vi "uTTA_Reset.vi"(4 "error in":errorcluster, 7 "uTTA Port":refnum<visa-resource-name>) -> (0 "error out":errorcluster, 3 "uTTA Port out":refnum<visa-resource-name>)   [LabVIEW 2021]
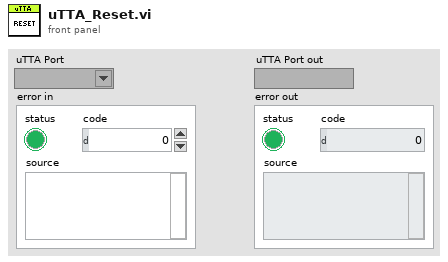
[diagram p1: front panel]
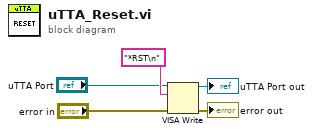
[diagram p0: block diagram]
diagram:
  n1 = VISA Write(VISA resource name="uTTA Port", write buffer="*RST\n", error in (no error)="error in") -> (VISA resource name out=→"uTTA Port out":refnum<visa-resource-name>, error out=→"error out":errorcluster)  [unwired: 1 out]
